vi "NI 5772 (AC) - TIS Mode Enabled (FPGA).vi"() -> ()   [LabVIEW 2015, in "DDC_7976R_v1.lvlib"]
doc: "Example Description:\nThis example demonstrates how to enable Time Interleaved Sampling with the NI 5772 adapter module to achieve a sampling rate of 1.6GS/s. This example continuously acquires records of analog input data from the NI 5772 adapter module. It allows you to select an AI channel, trigger type, and record size. This VI must be compiled before it is run. \n\nRunning the VI:\nThis VI must be run from the NI 5772 - Getting Started (Host).vi. Refer to the host VI documentation for steps regarding running and configuring the FPGA VI. \n\nExecution Steps:\nRefer to the Block Diagram of this VI for execution comments."
uses:
  DDC_7976R_v1.lvlib
  <instrlib>/_niInstr/DSP/v1/Shared/Public/IQ Gain.ctl
  <instrlib>/_niInstr/DSP/v1/Shared/Public/IQ Data.ctl
  <vilib>/Platform/TimedLoop/XDataNode/timing_clust.ctl
  <vilib>/Platform/TimedLoop/XDataNode/nitl_modes.ctl
  <vilib>/Platform/TimedLoop/XDataNode/wakeup.ctl
  <vilib>/rvi/Emulation/niFpgaGetClockAttributes.vi
  <vilib>/rvi/Emulation/niFpgaSctlEmulationGetInTimedLoop.vi
  <vilib>/rvi/Emulation/niFpgaEmulationReportErrorSimple.vi
  <vilib>/rvi/eio/common/nirviEmuTemplateMethod_errors.vi
  <vilib>/rvi/Emulation/niFpgaCriticalErrorInLSC.vi
  <vilib>/rvi/interface/RandomDataEmulation/nirviRandomDataMultiElementFPGAFIFO.vi
  <instcachedir>/0/nirviRandomDataMultiElementFPGAFIFO_8F99493546E24284B0D6A8E519C457F7.lvgen/nirviRandomDataMultiElementFPGAFIFO_8F99493546E24284B0D6A8E519C457F7_003.vi
  <vilib>/rvi/interface/RandomDataEmulation/niFpgaRandomDataHandleErrors.vi
  <instrlib>/_niInstr/DSP/v1/FPGA/Public/Sub VIs/Frequency Shift/Frequency Shift - 8 spc.vi
  <instrlib>/_niInstr/DSP/v1/FPGA/Public/Sub VIs/Digital Gain/Digital Gain Base.vi
  <instrlib>/_niInstr/DSP/v1/FPGA/Public/Sub VIs/Fractional Decimator/Fractional Decimator - 8 spc - 2x oc.vi
  <vilib>/eio/EIONode/EIONode.xnode
  <vilib>/Platform/TimedLoop/XDataNode/XDataNode.xnode
  <vilib>/rvi/DataTransferAndStorage/Container/XNode/niFpgaContainer.xnode
  <vilib>/rvi/interface/RandomDataEmulation/nirviRandomDataFpgaMultiElementTemplate.vi
  <instrlib>/_niInstr/DSP/v1/Xnodes/Public/Frequency Shift/niInstr DSP v1 Frequency Shift FPGA.xnode
  <instrlib>/_niInstr/DSP/v1/Xnodes/Public/Digital Gain/niInstr DSP v1 Digital Gain FPGA.xnode
  <instrlib>/_niInstr/DSP/v1/Xnodes/Public/Decimator/niInstr DSP v1 Decimator FPGA.xnode
  <vilib>/Platform/TimedLoop/XDataNode/XDNodeRunTimeDep.lvlib
  <instrlib>/_niInstr/DSP/v1/Shared/niInstr DSP v1 Shared.lvlib
  <instrlib>/_niInstr/DSP/v1/FPGA/niInstr DSP v1 FPGA.lvlib
  <instrlib>/_niInstr/Basic Elements/v1/FPGA/niInstr Basic Elements v1 FPGA.lvlib
panel:
  out "Array":u32[](array[numeric])
  out "data out":T1[](array[typedef])
  out "input saples":T1[](array[typedef])
  out "ver.editorial":u8
  out "ver.technical":u8=1
  out "ver.major":u8=1
  in  "trig.samples.to.acq":u64
  in  "mode.continuous":bool
  out "dma.overflow":bool
  out "dsp.overflow":bool
  in  "output sample rate":fxp<+,48,1>
  in  "delay":fxp<+/-,16,0>
  in  "gain":T2={"gain I"=1.0, "gain Q"=1.0}
  in  "frequency shift":fxp<+/-,48,0>
  in  "acq.abort":bool
  in  "trig.sw start trigger":bool
  in  "acq.initiate":bool
  in  "acq.reset":bool
  in  "User Command Commit":bool
  in  "User Command":u8
  out "User Command Idle":bool
  out "User Command Status":u8
  in  "User Data 0":u16
  in  "User Data 1":u8
  out "PLL Locked":bool
  out "User Error":bool
  out "Configured?":bool
  # "Resource Configuration"
  # "Refer to the Block Diagram of this VI for execution comments."
  # "For other instructions, select Help>>Show Context Help and move the cursor over the VI icon to display help for this VI."
  # "Analog Input"
  # "Clock Configuration"
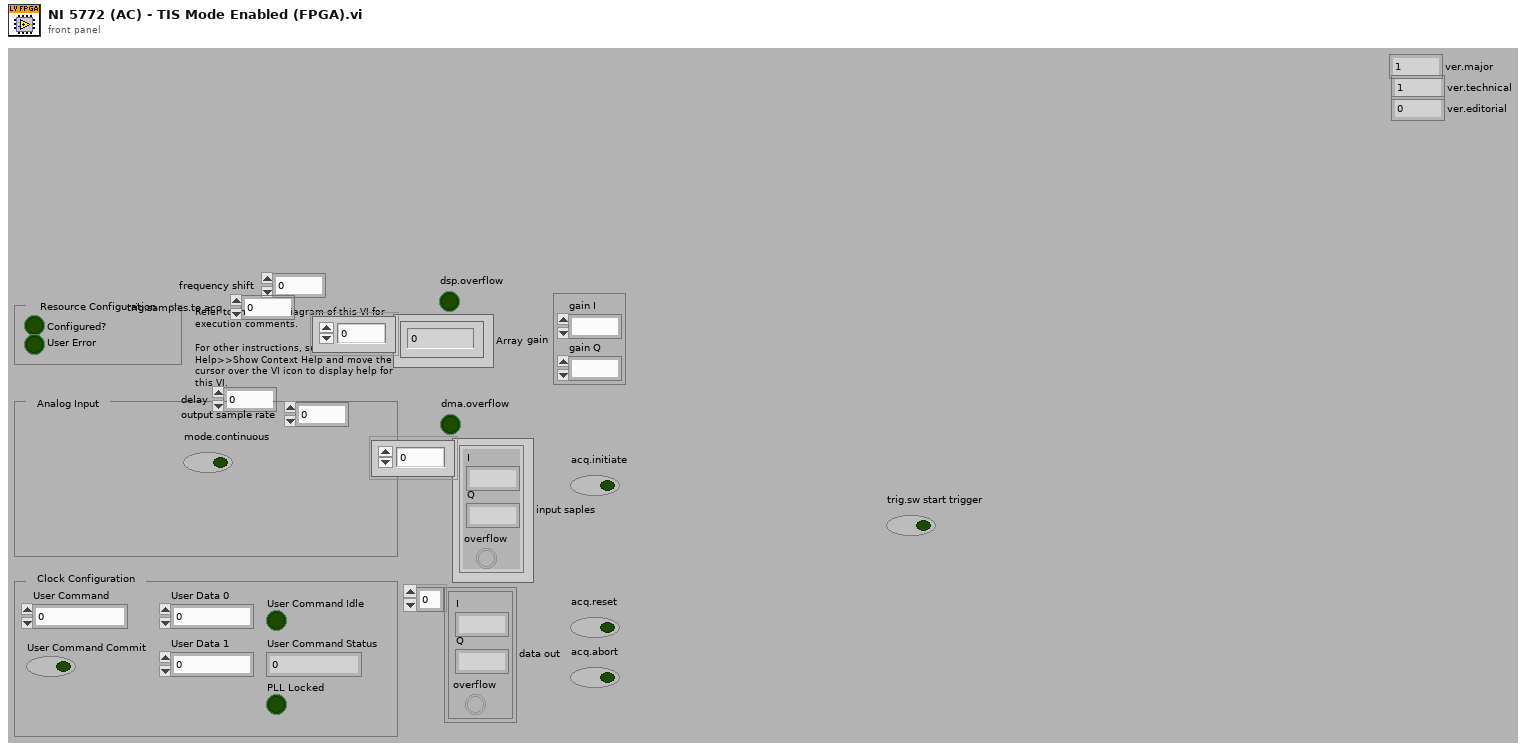
[diagram p1: front panel]
types:
  T1 = typedef "niInstr DSP v1 Shared.lvlib/IQ Data.ctl" = cluster{"I":fxp<+/-,18,1>, "Q":fxp<+/-,18,1>, "overflow":bool}
  T2 = typedef "niInstr DSP v1 Shared.lvlib/IQ Gain.ctl" = cluster{"gain I":fxp<+/-,24,3>, "gain Q":fxp<+/-,24,3>}
  T3 = typedef "XDNodeRunTimeDep.lvlib/timing_clust.ctl" = cluster{"Expected End [f-1]":u64, "Actual End [f-1]":u64, "Finished Late? [f-1]":bool, "Expected End [i-1]":u64, "Actual End [i-1]":u64, "Finished Late? [i-1]":bool, "Expected Start [i]":u64, "Actual Start [i]":u64, "Expected Start [f]":u64, "Actual Start [f]":u64, "Source Name":string, "Structure Name":string, "Period":i64, "Deadline":i64, "Offset":i64, "Start":i64, "Priority":i32, "Timeout":i32, "Mode":T4, "Wakeup Reason":T5, "Error":errorcluster, "Source Type":string, "Secondary Source Type":string, "Global End Time":u64, "Global Start Time":u64, "Frame Duration":u64, "Iteration Duration":u64, "Assigned CPU":i32, "I/O Scan Engine Mode":u32}
  T4 = typedef "XDNodeRunTimeDep.lvlib/nitl_modes.ctl" = enum32{"No Change", "Process missed periods, maintain original phase", "Discard missed periods, maintain original phase", "Process missed periods, ignore original phase", "Discard missed periods, ignore original phase"}
  T5 = typedef "XDNodeRunTimeDep.lvlib/wakeup.ctl" = enum32{"Normal", "Aborted", "Asynchronous wakeup", "Timing source error", "Timed loop error", "Timeout"}
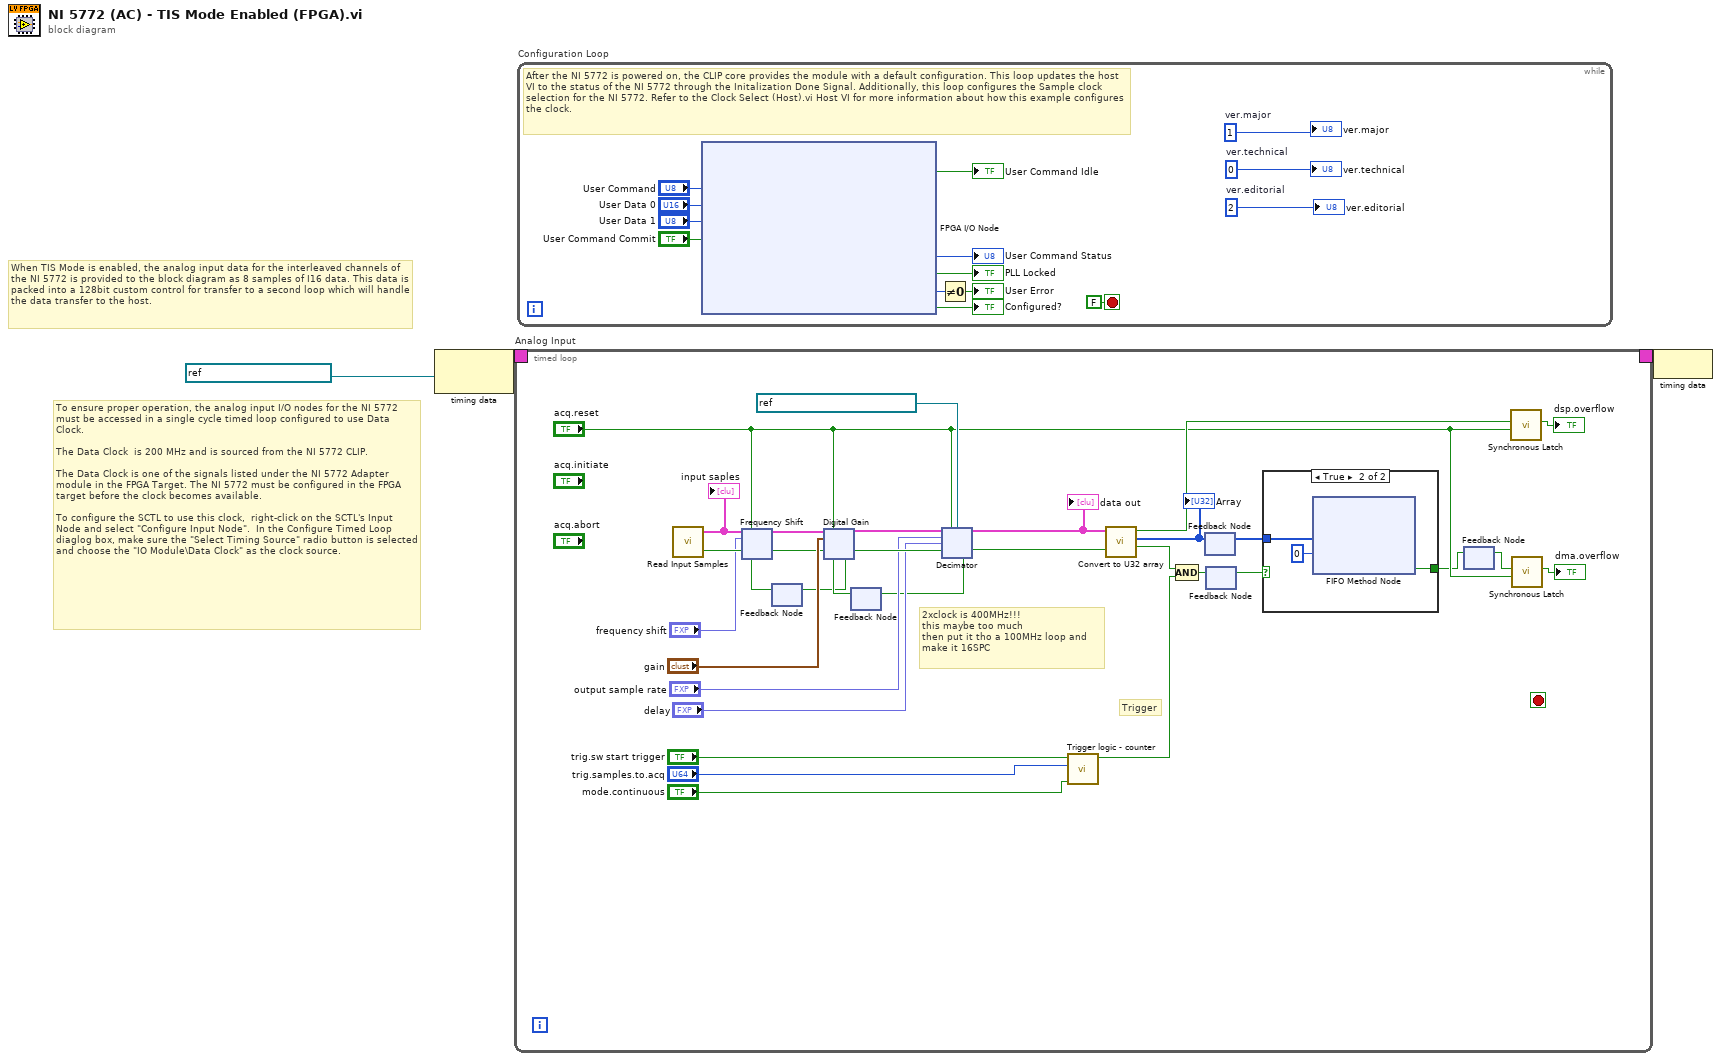
[diagram p0: block diagram]
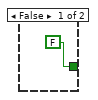
[diagram p2: hidden frame]
diagram:
  # "When TIS Mode is enabled, the analog input data for the interleaved channels of the NI 5772 is provided to the block diagram as 8 samples of I16 data. This data is packed into a 128bit custom control for transfer to a second loop which will handle the data transfer to the host."
  # "To ensure proper operation, the analog input I/O nodes for the NI 5772 must be accessed in a single cycle timed loop configured to use Data Clock. \n\nThe Data Clock  is 200 MHz and is sourced from the NI 5772 CLIP.\n\nThe Data Clock is one of the signals listed under the NI 5772 Adapter module in the FPGA Target. The NI 5772 must be configured in the FPGA target before the clock becomes available. \n\nTo configure the SCTL to use this clock,  right-click on the SCTL's Input Node and select \"Configure Input Node\".  In the Configure Timed Loop diaglog box, make sure the \"Select Timing Source\" radio button is selected and choose the \"IO Module\\Data Clock\" as the clock source."
  n1 = node-c288(refnum<k21> "IO Module\\Data Clock" ("Source Name")) -> (w3:T3)
  n2 = timed-loop "Analog Input" {
    timing: w3 -> [_]
    timing-out: [_] -> w2
    stop <- _ stop-if-true
    # "2xclock is 400MHz!!!\nthis maybe too much\nthen put it tho a 100MHz loop and\nmake it 16SPC"
    # "Trigger"
    n3 = call "Read Input Samples.vi"() -> ("Array"=w35:T1[], "output valid"=w33:bool)  [unwired: 14 in]
    "input saples" <- w35
    n4 = feedback #1() -> (w21:bool)  [unwired: 1 in]
    n5 = xnode "Frequency Shift"("data in"=w35, "reset"="acq.reset", "frequency shift"="frequency shift", "input valid"=w33, "ready for output (T)"=w21) -> ("data out"=w34:T1[], "output valid"=w28:bool)  [unwired: 1 in, 1 out]
    n6 = feedback #2() -> (w23:bool)  [unwired: 1 in]
    n7 = xnode "Digital Gain"("data in"=w34, "reset"="acq.reset", "gain"="gain", "input valid"=w28, "ready for output (T)"=w23) -> ("data out"=w32:T1[], "output valid"=w27:bool, "ready for input"=w22:bool)
    n8 = feedback-in #1(w22) -> ()
    n9 = xnode "Decimator"("data in"=w32, "reset"="acq.reset", "input valid"=w27, "output sample rate"="output sample rate", "delay"="delay", "clock x2"=refnum<k21> "IO Module\\Data Clock 2x" ("Source Name")) -> ("data out"=w19:T1[], "output valid"=w8:bool, "ready for input"=w24:bool)  [unwired: 1 out]
    "data out" <- w19
    n10 = feedback-in #2(w24) -> ()
    n11 = call "Trigger logic - counter.vi"("mode.continuous"="mode.continuous", "trig.samples.to.acq"="trig.samples.to.acq", "trig.sw start trigger"="trig.sw start trigger") -> ("enable out"=w4:bool)  [unwired: 8 in]
    n12 = call "Convert to U32 array.vi"("input valid"=w8, "data in"=w19) -> ("output valid"=w15:bool, "Array"=w14:u32[], "overflow"=w18:bool)  [unwired: 7 in]
    "Array" <- w14
    n13 = Compound Arithmetic op=AND(w15, w4) -> (w12:bool)
    n14 = feedback #3() -> (w13:u32[])  [unwired: 1 in]
    n15 = feedback-in #3(w14) -> ()
    n16 = feedback #4() -> (w11:bool)  [unwired: 1 in]
    n17 = feedback-in #4(w12) -> ()
    n18 = case shown="True" w11 {
      tunnel: w13 -> [_ w39]
      tunnel: [FALSE ("Timed Out?") w37] -> w10
      frame False {
      }
      frame True {
        n19 = xnode ("FIFO Method Node")("Element"=w39, "Timeout"=0) -> ("Timed Out?"=w37:bool)  [unwired: 1 in, 1 out]
      }
    }
    n20 = feedback #5() -> (w9:bool)  [unwired: 1 in]
    n21 = feedback-in #5(w10) -> ()
    n22 = call <instrlib>:"Synchronous Latch.vi"("clear"="acq.reset", "set"=w18) -> ("out"=→"dsp.overflow":bool)  [unwired: 9 in]
    n23 = call <instrlib>:"Synchronous Latch.vi"("clear"="acq.reset", "set"=w9) -> ("out"=→"dma.overflow":bool)  [unwired: 9 in]
  }
  n24 = while "Configuration Loop" {
    stop <- FALSE stop-if-true
    w100 = u8 2  # ver.editorial
    w101 = u8 0  # ver.technical
    w102 = u8 1  # ver.major
    # "After the NI 5772 is powered on, the CLIP core provides the module with a default configuration. This loop updates the host VI to the status of the NI 5772 through the Initalization Done Signal. Additionally, this loop configures the Sample clock selection for the NI 5772. Refer to the Clock Select (Host).vi Host VI for more information about how this example configures the clock."
    n25 = xnode "FPGA I/O Node"("IO Module\\User Command"="User Command", "IO Module\\User Data 0"="User Data 0", "IO Module\\User Data 1"="User Data 1", "IO Module\\User Command Commit"="User Command Commit") -> ("IO Module\\User Command Idle"=→"User Command Idle":bool, "IO Module\\User Command Status"=→"User Command Status":u8, "IO Module\\PLL Locked"=→"PLL Locked":bool, "IO Module\\User Error"=w108:u8, "IO Module\\Initialization Done"=→"Configured?":bool)  [unwired: 9 in, 9 out]
    n26 = Not Equal To 0?(x=w108) -> (x != 0?=→"User Error":bool)
    "ver.major" <- w102
    "ver.technical" <- w101
    "ver.editorial" <- w100
  }
  n27 = node-c288(w2) -> ()
